vi "EXA_ackCommand_SetValue.vi"(8 "error in (no error)":errorcluster, 11 "ackcmd_Ctl":T1={"cmdSeqNum"=0, "ack"=0, "error"=0, "result"="                                                                                                                                                                                                                                                                "}) -> (0 "error out":errorcluster, 2 "function return":i32, 3 "ackcmd_Ctl out":T1={"cmdSeqNum"=0, "ack"=0, "error"=0, "result"="                                                                                                                                                                                                                                                                "})   [LabVIEW 2016, in "SALLV_EXA.lvlib"]
doc: "int EXA_shm_ackCommand_SetValueLV(EXA_ackcmdLV *ackcmd_Ctl);"
uses:
  SALLV_EXA.lvlib
  DataTypes/ackcmd.ctl
  SALLV_EXA.so
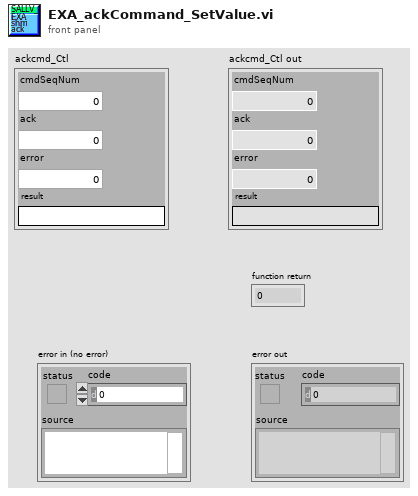
[diagram p1: front panel]
types:
  T1 = typedef "SALLV_EXA.lvlib/ackcmd.ctl" = cluster{"cmdSeqNum":i32, "ack":i32, "error":i32, "result":string}
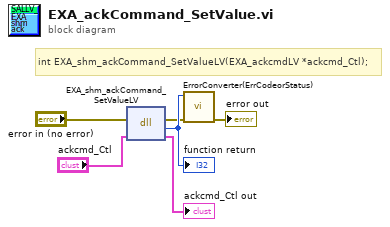
[diagram p0: block diagram]
diagram:
  # "int EXA_shm_ackCommand_SetValueLV(EXA_ackcmdLV *ackcmd_Ctl);"
  n1 = dll-call lib="home/andres/Desktop/EXA_SAL_LV/SALLV_EXA.*" fn="EXA_shm_ackCommand_SetValueLV"(error in="error in (no error)", "ackcmd_Ctl"="ackcmd_Ctl") -> (error out=w2:errorcluster, w6:i32, "ackcmd_Ctl"=→"ackcmd_Ctl out":T1)  [unwired: 2 in, 1 out]
  "function return" <- w6
  n2 = call "ErrorConverter(ErrCodeorStatus).vi"("error in (no error)"=w2, "error code"=w6) -> ("error out"=→"error out":errorcluster)  [unwired: 9 in]
